vi "Read Active State.vi"(8 "error in (no error)":errorcluster, 11 "Command Processor in":refnum<class "Command Processor.lvclass">) -> (0 "error out":errorcluster, 2 "Active State":string, 3 "Command Processor out":refnum<class "Command Processor.lvclass">)   [LabVIEW 2013, in "Command Processor.lvlib" / "Command Processor.lvclass"]
uses:
  Command Processor.lvclass
  Command Processor.lvclass/Command Processor.ctl
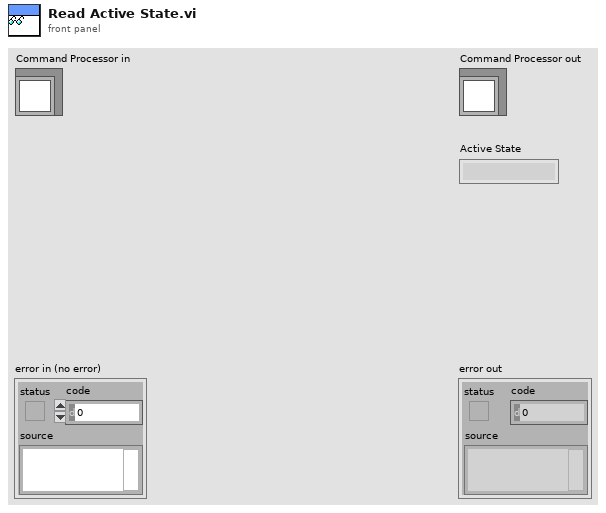
[diagram p1: front panel]
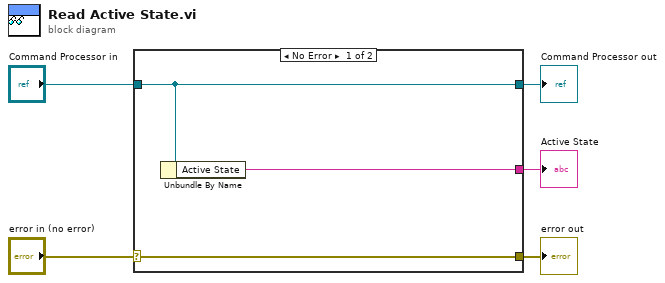
[diagram p0: block diagram]
diagram:
  n1 = case shown="No Error" "error in (no error)" {
    selector: "error in (no error)" -> [w8 w9]
    tunnel: [w8 w9] -> w4
    tunnel: [w7 w10] -> w2
    tunnel: "Command Processor in" -> [w7 w10]
    tunnel: [w6 _] -> w1
    frame No Error {
      n2 = Unbundle By Name(w7) -> ("Active State"=w6:string)
    }
    frame Error {
    }
  }
  "error out" <- w4
  "Command Processor out" <- w2
  "Active State" <- w1
